vi "Send Generate Event.vi"(7 "Message Priority (Normal)":T1=enum."Normal", 8 "error in":errorcluster, 9 "Event Data":refnum<class "Event Data.lvclass">, 10 "Event Name":string, 11 "Message Enqueuer":refnum<class "Message Enqueuer.lvclass">) -> (0 "error out":errorcluster, 3 "Message Enqueuer out":refnum<class "Message Enqueuer.lvclass">)   [LabVIEW 2021, in "EventSourceActor.lvlib" / "Event Source.lvlib" / "Generate Event Msg.lvclass"]
doc: "This VI sends the message to an actor."
uses:
  Generate Event Msg.lvclass
  <vilib>/ActorFramework/Message Enqueuer/Message Enqueuer.lvclass
  <vilib>/ActorFramework/Message Enqueuer/Message Priority.ctl
  Event Data/Event Data.lvclass
  C:/Program Files/National Instruments/LabVIEW 2021/vi.lib/ActorFramework/Message/Message.lvclass
  Generate Event Msg.lvclass/Generate Event Msg.ctl
  <vilib>/ActorFramework/Message Enqueuer/Message Enqueuer.lvclass/Message Enqueuer.ctl
  <vilib>/ActorFramework/Message Priority Queue/Priority Enqueue.vi
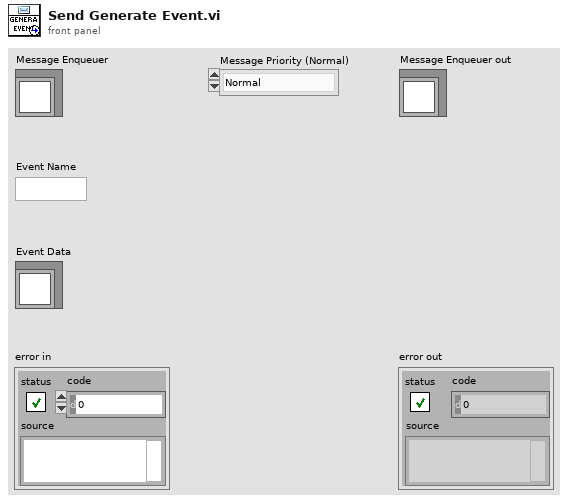
[diagram p1: front panel]
types:
  T1 = typedef "Actor Framework.lvlib/Message Enqueuer.lvclass/Message Priority.ctl" = enum16{"Low", "Normal", "High"}
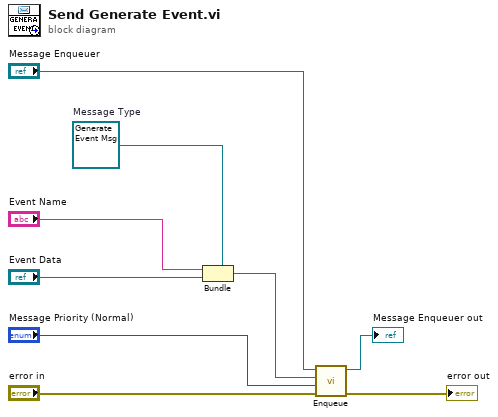
[diagram p0: block diagram]
diagram:
  w6 = refnum<class "Generate Event Msg.lvclass"> refnum  # Message Type
  n1 = Bundle(cluster=w6, "Event Name", "Event Data") -> (w5:refnum<class "Generate Event Msg.lvclass">)
  n2 = call <vilib>:"Enqueue.vi"("error in (no error)"="error in", "Message Priority (Normal)"="Message Priority (Normal)", "Message"=w5, "Message Enqueuer in"="Message Enqueuer") -> ("error out"=→"error out":errorcluster, "Message Enqueuer out"=→"Message Enqueuer out":refnum<class "Message Enqueuer.lvclass">)  [unwired: 6 in]
